vi "CallConvert.vi"(7 "Close?":bool, 8 "error in (no error)":errorcluster) -> (0 "error out":errorcluster, 1 "SRList":T1 {"SR#" format="%#_10g"}, 2 "DataValid?":bool)   [LabVIEW 2017, in "Server.lvlib" / "Oracle.lvlib"]
doc: "This VI will call a VI asynchronuously if its not already running. If its running it will poll if it finished and output the data."
uses:
  Oracle.lvlib
  TypeDefs/SR List.ctl
  TypeDefs/SR Data.ctl
  Server.lvlib
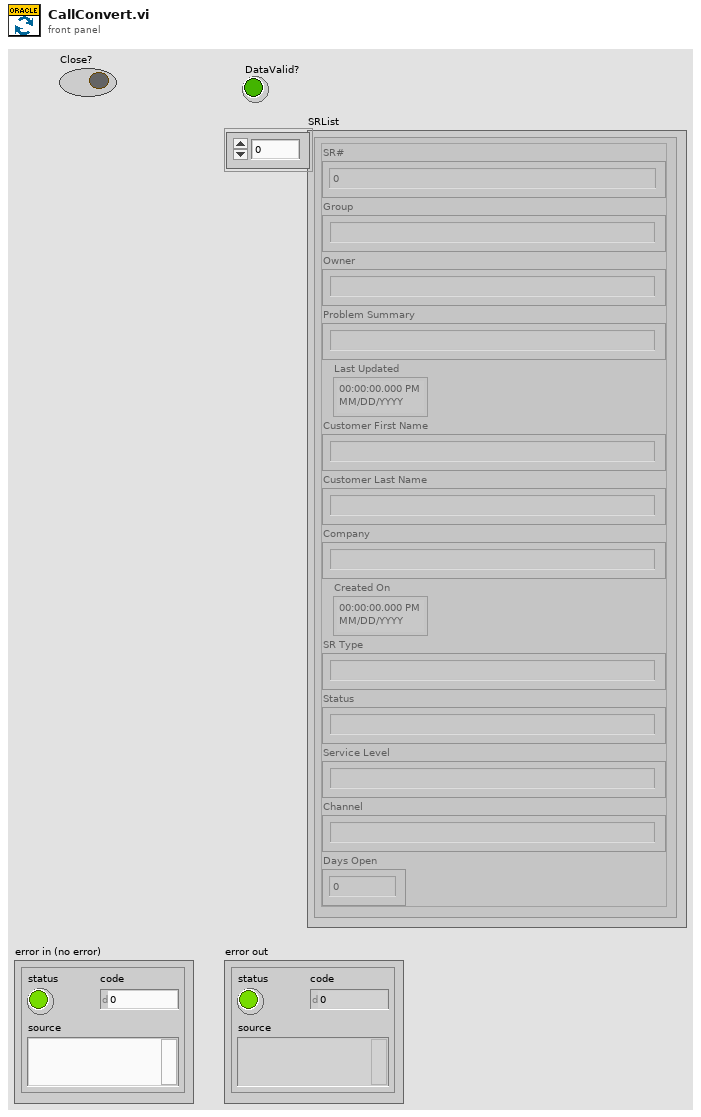
[diagram p1: front panel]
types:
  T1 = typedef "Server.lvlib/SR List.ctl" = T2[]
  T2 = typedef "Server.lvlib/SR Data.ctl" = cluster{"SR#":dbl, "Group":string, "Owner":string, "Problem Summary":string, "Last Updated":timestamp, "Customer First Name":string, "Customer Last Name":string, "Company":string, "Created On":timestamp, "SR Type":string, "Status":string, "Service Level":string, "Channel":string, "Days Open":dbl}
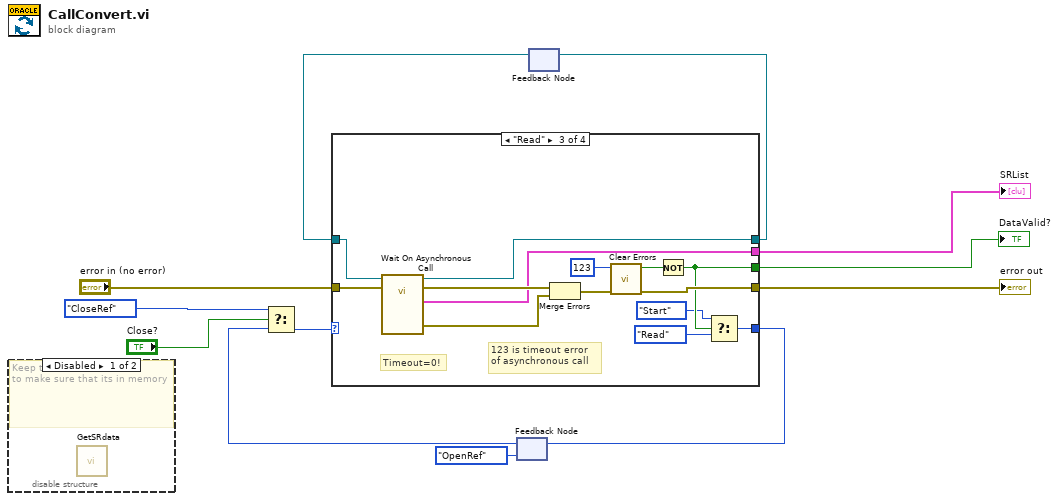
[diagram p0: block diagram]
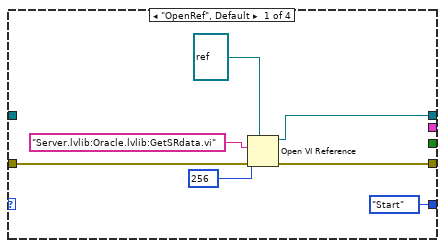
[diagram p2: hidden frame]
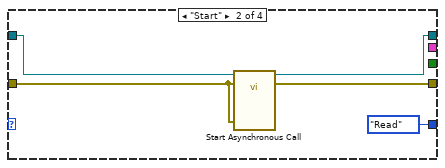
[diagram p3: hidden frame]
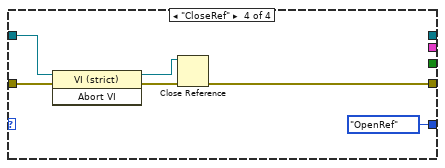
[diagram p4: hidden frame]
diagram:
  n1 = disable-structure shown="Disabled" {
    frame Disabled {
      # "Keep this VI here disabled \nto make sure that its in memory"
      n2 = call "GetSRdata.vi"() -> ()  [unwired: 10 in, 2 out]
    }
    frame Enabled {
    }
  }
  n3 = feedback #1(enum16{"OpenRef", "Start", "Read", "CloseRef"}."OpenRef") -> (w7:enum16{"OpenRef", "Start", "Read", "CloseRef"})
  n4 = Select(t=enum16{"OpenRef", "Start", "Read", "CloseRef"}."CloseRef", s="Close?", f=w7) -> (s? t:f=w3:enum16{"OpenRef", "Start", "Read", "CloseRef"})
  n5 = feedback #2() -> (w5:refnum<vi>)  [unwired: 1 in]
  n6 = case shown="\"Read\"" w3 {
    tunnel: [w18 w24 w32 w40] -> w11
    tunnel: "error in (no error)" -> [w19 w23 w38 w44]
    tunnel: [w14 w22 w31 _] -> w6
    tunnel: [_ _ w33 _] -> w10
    tunnel: [_ _ w28 _] -> w12
    tunnel: [enum16{"OpenRef", "Start", "Read", "CloseRef"}."Start" enum16{"OpenRef", "Start", "Read", "CloseRef"}."Read" w25 enum16{"OpenRef", "Start", "Read", "CloseRef"}."OpenRef" ("t")] -> w8
    tunnel: w5 -> [_ w21 w29 w41]
    frame "OpenRef", Default {
      n7 = Open VI Reference(type specifier VI Refnum (for type only)=refnum<vi> refnum, vi path="Server.lvlib:Oracle.lvlib:GetSRdata.vi", options=256, error in (no error)=w19) -> (vi reference=w14:refnum<vi>, error out=w18:errorcluster)  [unwired: 2 in]
    }
    frame "Start" {
      n8 = call-by-ref "Start Asynchronous Call"(reference=w21, error in=w23, "Error In"=w23) -> (reference out=w22:refnum<vi>, error out=w24:errorcluster)  [unwired: 9 in, 2 out]
    }
    frame "Read" {
      # "123 is timeout error\nof asynchronous call"
      # "Timeout=0!"
      n9 = call-by-ref "Wait On Asynchronous Call"(reference=w29, error in=w38) -> (reference out=w31:refnum<vi>, error out=w37:errorcluster, "Error Out"=w34:errorcluster, "SRList"=w33:T1)  [unwired: 10 in]
      n10 = Merge Errors(w37, w34) -> (w35:errorcluster)
      n11 = call <vilib>:"Clear Errors.vi"("error in (no error)"=w35, "specific error code to clear (0: all)"=123) -> ("error out"=w32:errorcluster, "specific error cleared?"=w30:bool)  [unwired: 4 in]
      n12 = Not(x=w30) -> (.not. x?=w28:bool)
      n13 = Select(t=enum16{"OpenRef", "Start", "Read", "CloseRef"}."Start", s=w28, f=enum16{"OpenRef", "Start", "Read", "CloseRef"}."Read") -> (s? t:f=w25:enum16{"OpenRef", "Start", "Read", "CloseRef"})
    }
    frame "CloseRef" {
      n14 = invoke class="VI (strict)" method="Abort VI"(reference=w41, error in=w44) -> (reference out=w39:refnum<vi>, error out=w42:errorcluster)  [unwired: 1 in, 1 out]
      n15 = Close Reference(reference=w39, error in (no error)=w42) -> (error out=w40:errorcluster)
    }
  }
  "DataValid?" <- w12
  "error out" <- w11
  "SRList" <- w10
  n16 = feedback-in #1(w8) -> ()
  n17 = feedback-in #2(w6) -> ()
